vi "Test Weight Grab and Replace.vi"() -> ()   [LabVIEW 2011]
uses:
  Gantry Class/Gantry Class.lvclass
  CameraTool Class/CameraTool Class.lvclass
  Config Manager Class/Type Definitions/Fiducial Type.ctl
  CameraTool Class/Type Definitions/Fiducial Acquisition Parameters.ctl
  Config Manager Class/Config Manager Class.lvclass
  GrabberTool Class.lvclass
  Orient3d Class/Orient3d Class.lvclass
  Vec3d Class/Vec3d Class.lvclass
  Utils/Type Definitions/Position_Orientation.ctl
  WorkTable Class/WorkTable Class.lvclass
  Config Manager Class/Type Definitions/Weight Type.ctl
  WorkTable Class/Type Definitions/Worktable_Weight.ctl
panel:
  in  "Weight Slot":i32
  in  "Virtual Mode":bool
  out "error out":errorcluster
  in  "Config Folder":path=path "C:/Users/husker/Desktop/gantry/Config"
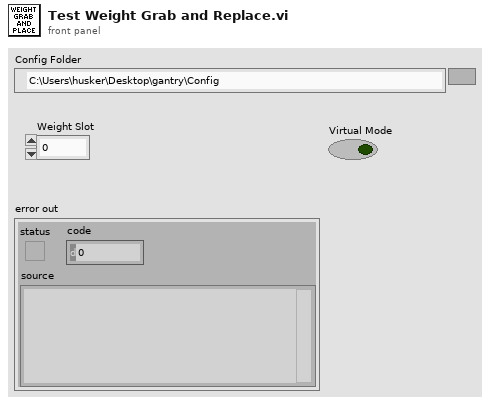
[diagram p1: front panel]
types:
  T1 = typedef "Worktable_Weight.ctl" = cluster{"Weight State":enum16{"Empty", "Populated"}, "Weight Type":T2, "Location/Orientation":T3}
  T2 = typedef "Weight Type.ctl" = enum16{"Weight 1", "Weight 2", "Weight 3", "Weight 4", "Weight 5", "Weight 6", "Weight 7", "Weight 8"}
  T3 = typedef "Position_Orientation.ctl" = cluster{"Center":refnum<class "Vec3d Class.lvclass">, "Orientation":refnum<class "Orient3d Class.lvclass">}
  T4 = typedef "Fiducial Type.ctl" = enum16{"HDI", "BBM"}
  T5 = typedef "Fiducial Acquisition Parameters.ctl" = cluster{"Selection Criteria":enum16{"Single", "Top", "Bottom"}, "Image Prefix":string, "Fiducial Type":T4}
  T6 = cluster{"Feature Coordinates":refnum<class "Vec3d Class.lvclass">, "Feature Name":string}[]
  T7 = typedef "Fiducial Image.ctl" = cluster{"Fiducial Image":T8, "Selected Fiducial":T10, "fiducial name":string}
  T8 = typedef "Physical Image.ctl" = cluster{"Image Position":refnum<class "Vec3d Class.lvclass">, "Image Reference":T9, "Field of View":cluster{"x(mm)":dbl, "y(mm)":dbl}}
  T9 = typedef "IMAQ Image.ctl" = refnum<image>
  T10 = typedef "Fiducial with Source.ctl" = cluster{"Fiducial Image Coordinate":refnum<class "Vec3d Class.lvclass">, "Fiducial Source":enum16{"Pattern Recognition", "User", "Error", "Default"}}
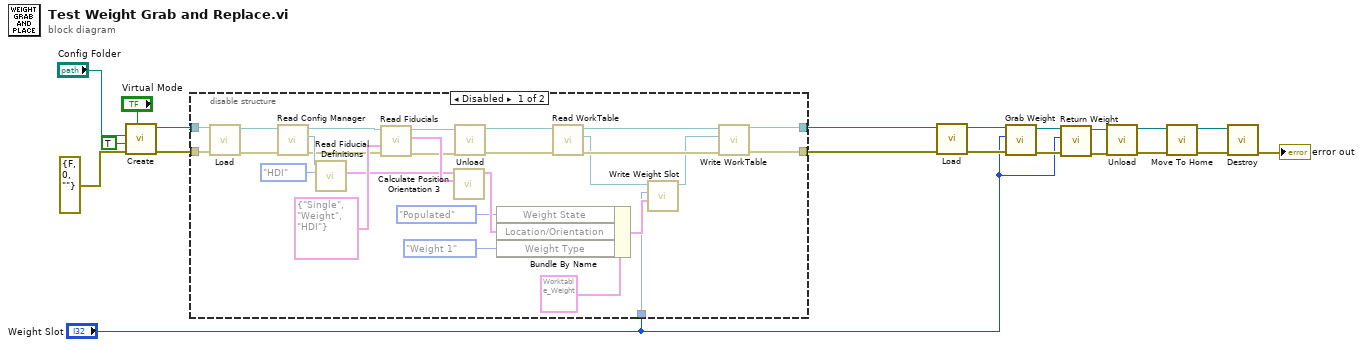
[diagram p0: block diagram]
diagram:
  n1 = call "Create.vi"("Virtual Mode"="Virtual Mode", "error in"=errorcluster {"status"=FALSE, "code"=0, "source"=""}, "HOME?"=TRUE, "Config Folder"="Config Folder") -> ("error out"=w18:errorcluster, "Gantry out"=w19:refnum<class "Gantry Class.lvclass">)  [unwired: 6 in]
  n2 = disable-structure shown="Disabled" {
    disable-tunnel: w19 -> [w47 w49]
    disable-tunnel: w18 -> [w36 w48]
    disable-tunnel: [w27 w49] -> w7
    disable-tunnel: [w26 w48] -> w6
    disable-tunnel: "Weight Slot" -> [w21 _]
    frame Disabled {
      n3 = call "Load.vi"("error in"=w36, "Gantry In"=w47) -> ("error out"=w35:errorcluster, "CameraTool out"=w42:refnum<class "CameraTool Class.lvclass">)  [unwired: 8 in]
      n4 = call-dynamic "Read Config Manager.vi"("error in"=w35, "Gantry in"=w42) -> ("error out"=w34:errorcluster, "Config Manager"=w41:refnum<class "Config Manager Class.lvclass">, "Gantry out"=w40:refnum<class "CameraTool Class.lvclass">)  [unwired: 7 in]
      n5 = call "Read Fiducial Definitions.vi"("Fiducial Type"=Fiducial_Type."HDI", "Config Manager in"=w41) -> ("Feature Definitions"=w44:T6)  [unwired: 7 in, 2 out]
      n6 = call-dynamic "Read Fiducials.vi"("error in"=w34, "Fiducial Acquisition Parameters"=T5 {"Selection Criteria"=enum."Single", "Image Prefix"="Weight", "Fiducial Type"=enum."HDI"}, "CameraTool in"=w40) -> ("error out"=w33:errorcluster, "Fiducials"=w45:T7[], "CameraTool out"=w39:refnum<class "CameraTool Class.lvclass">)  [unwired: 6 in]
      n7 = call "Calculate Position Orientation 3.vi"("Fiducials"=w45, "Feature Definitions"=w44) -> ("PositionOrientation"=w37:T3)  [unwired: 8 in, 1 out]
      n8 = call "Unload.vi"("error in"=w33, "CameraTool in"=w39) -> ("error out"=w24:errorcluster, "Gantry out"=w25:refnum<class "Gantry Class.lvclass">)  [unwired: 8 in]
      n9 = Bundle By Name(cluster=T1 {"Weight State"=enum."Empty", "Weight Type"=enum."Weight 1", "Location/Orientation"={"Center"=refnum, "Orientation"=refnum}} ("Weight Slot"), "Weight State"=enum16{"Empty", "Populated"}."Populated", "Location/Orientation"=w37, "Weight Type"=Weight_Type."Weight 1") -> (w22:T1)
      n10 = call-dynamic "Read WorkTable.vi"("error in"=w24, "Gantry Class in"=w25) -> ("error out"=w32:errorcluster, "WorkTable Class.lvclass"=w31:refnum<class "WorkTable Class.lvclass">, "Gantry Class out"=w38:refnum<class "Gantry Class.lvclass">)  [unwired: 7 in]
      n11 = call "Write Weight Slot.vi"("Weight Slot"=w22, "weight slot"=w21, "WorkTable Class in"=w31) -> ("WorkTable Class out"=w30:refnum<class "WorkTable Class.lvclass">)  [unwired: 7 in, 1 out]
      n12 = call-dynamic "Write WorkTable.vi"("error in (no error)"=w32, "WorkTable Class.lvclass"=w30, "Gantry Class in"=w38) -> ("error out"=w26:errorcluster, "Gantry Class out"=w27:refnum<class "Gantry Class.lvclass">)  [unwired: 7 in]
    }
    frame Enabled {
    }
  }
  n13 = call "Load.vi"("error in"=w6, "Gantry In"=w7) -> ("error out"=w8:errorcluster, "Grabber Tool out"=w9:refnum<class "GrabberTool Class.lvclass">)  [unwired: 8 in]
  n14 = call "Grab Weight.vi"("error in"=w8, "Weight Number"="Weight Slot", "GrabberTool in"=w9) -> ("error out"=w14:errorcluster, "GrabberTool out"=w15:refnum<class "GrabberTool Class.lvclass">)  [unwired: 7 in]
  n15 = call "Return Weight.vi"("error in"=w14, "Slot Number"="Weight Slot", "GrabberTool in"=w15) -> ("error out"=w12:errorcluster, "GrabberTool out"=w13:refnum<class "GrabberTool Class.lvclass">)  [unwired: 7 in]
  n16 = call "Unload.vi"("error in"=w12, "GrabberTool in"=w13) -> ("error out"=w2:errorcluster, "Gantry out"=w4:refnum<class "Gantry Class.lvclass">)  [unwired: 8 in]
  n17 = call-dynamic "Move To Home.vi"("error in"=w2, "Gantry in"=w4) -> ("error out"=w1:errorcluster, "Gantry out"=w3:refnum<class "Gantry Class.lvclass">)  [unwired: 8 in]
  n18 = call "Destroy.vi"("error in"=w1, "Gantry Class in"=w3) -> ("error out"=→"error out":errorcluster)  [unwired: 9 in]
